vi "VSI Init SPI.vi"(8 "error in (no error)":errorcluster, 9 "pInitConfig":T1, 10 "DevIndex":i32, 11 "DevType":i32) -> (0 "error out":errorcluster, 3 "function return":i32)   [LabVIEW 2012, in "ControlSPI.lvlib"]
doc: "int WINAPI VSI_InitSPI(int DevType, int DevIndex, PVSI_INIT_CONFIG pInitConfig);"
uses:
  ControlSPI.lvlib
  Ginkgo_Driver.dll
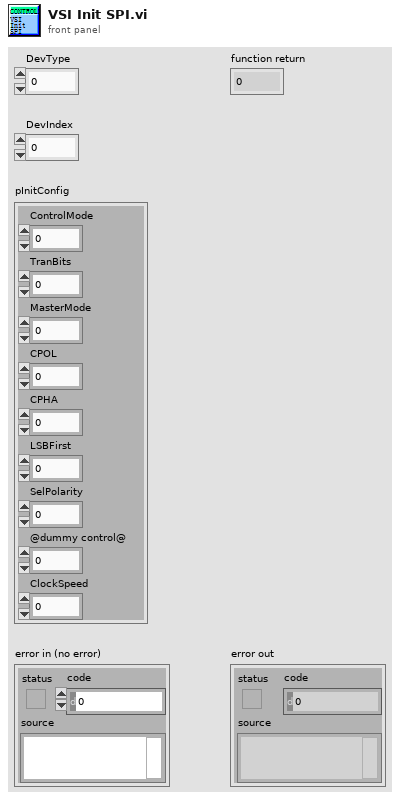
[diagram p1: front panel]
types:
  T1 = cluster{"ControlMode":u8, "TranBits":u8, "MasterMode":u8, "CPOL":u8, "CPHA":u8, "LSBFirst":u8, "SelPolarity":u8, "@dummy control@":i8, "ClockSpeed":u32}
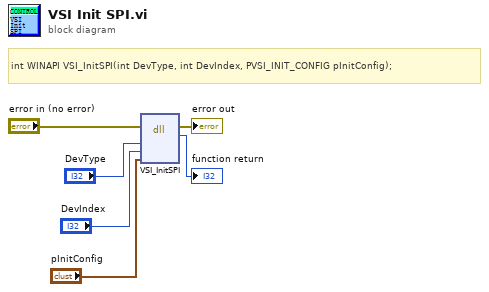
[diagram p0: block diagram]
diagram:
  # "int WINAPI VSI_InitSPI(int DevType, int DevIndex, PVSI_INIT_CONFIG pInitConfig);"
  n1 = dll-call lib="E:/Project/vt_ginkgo/truck/Ginkgo Driver/vs2010/Ginkgo_USB-I2C_API_v2.0.3.0/lib/labview_32bit/ControlSPI/Ginkgo_Driver.*" fn="VSI_InitSPI"(error in="error in (no error)", "DevType"="DevType", "DevIndex"="DevIndex", "pInitConfig"="pInitConfig") -> (error out=→"error out":errorcluster, →"function return":i32)  [unwired: 5 in, 1 out]
